vi "Read Calibration info.vi"(11 "Vector Network Analyzer in":refnum<class "Vector Network Analyzer.lvclass">) -> (2 "Calibration info":string, 3 "Vector Network Analyzer out":refnum<class "Vector Network Analyzer.lvclass">)   [LabVIEW 2020, in "Vector Network Analyzer.lvclass"]
uses:
  Vector Network Analyzer.lvclass
  Vector Network Analyzer.lvclass/Vector Network Analyzer.ctl
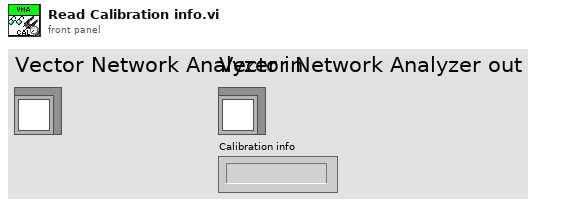
[diagram p1: front panel]
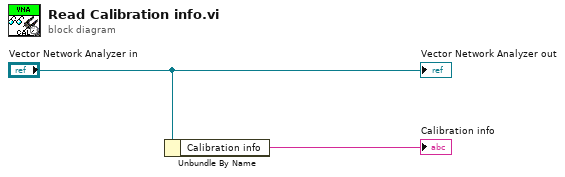
[diagram p0: block diagram]
diagram:
  n1 = Unbundle By Name("Vector Network Analyzer in") -> ("Calibration info"=→"Calibration info":string)
  "Vector Network Analyzer out" <- "Vector Network Analyzer in"
